vi "Type Query.vi"(8 "error in (no error)":errorcluster, 9 "Address (0)":i32, 11 "VISA resource name":refnum<visa-resource-name>) -> (0 "error out":errorcluster, 2 "Chamber Type":T1, 3 "VISA resource name out":refnum<visa-resource-name>)   [LabVIEW 2016, in "Environment Chamber.lvlib" / "Climatic Chamber.lvlib"]
doc: "<b>Chamber type monitor</B>\n\nReturns the type of sensor connected to the temperature controller, the type of temperature controller, and the set temperature upper limit."
uses:
  Climatic Chamber.lvlib
  Private/Type Defs/Chamber Type Cluster.ctl
  Private/Type Defs/Sensor Type Enum.ctl
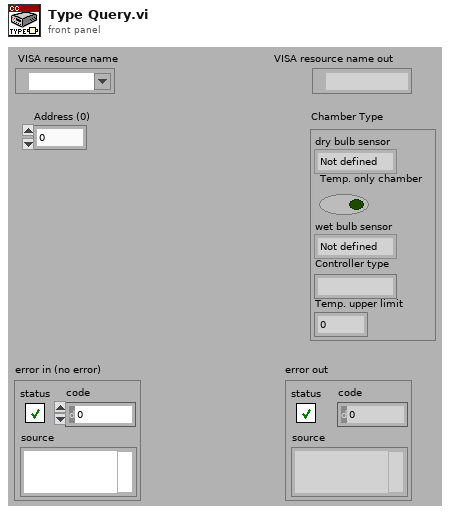
[diagram p1: front panel]
types:
  T1 = typedef "Environment Chamber.lvlib/Climatic Chamber.lvlib/Chamber Type Cluster.ctl" = cluster{"dry bulb sensor":T2, "Temp. only chamber":bool, "wet bulb sensor":T2, "Controller type":string, "Temp. upper limit":dbl}
  T2 = typedef "Environment Chamber.lvlib/Climatic Chamber.lvlib/Sensor Type Enum.ctl" = enum16{"Not defined", "Thermocouple"}
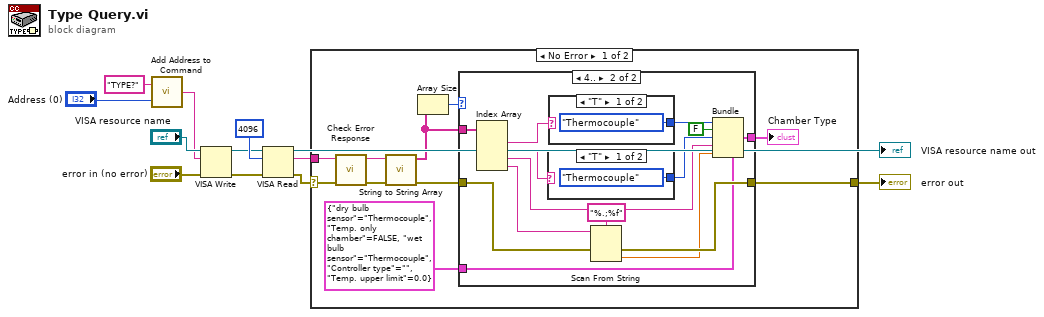
[diagram p0: block diagram]
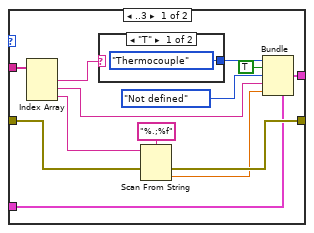
[diagram p2: hidden frame]
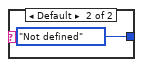
[diagram p3: hidden frame]
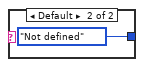
[diagram p4: hidden frame]
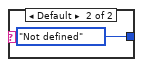
[diagram p5: hidden frame]
diagram:
  n1 = call "Add Address to Command.vi"("Address (0)"="Address (0)", "Command"="TYPE?") -> ("Command OUT"=w6:string)
  n2 = VISA Write(VISA resource name="VISA resource name", write buffer=w6, error in (no error)="error in (no error)") -> (VISA resource name out=w10:refnum<visa-resource-name>, error out=w9:errorcluster)  [unwired: 1 out]
  n3 = VISA Read(VISA resource name=w10, byte count=u32 4096 ("Bytes to Read"), error in (no error)=w9) -> (VISA resource name out=→"VISA resource name out":refnum<visa-resource-name>, read buffer=w3:string, error out=w2:errorcluster)  [unwired: 1 out]
  n4 = case shown="No Error" w2 {
    selector: w2 -> [w21 w56]
    tunnel: w3 -> [w22 _]
    tunnel: [w14 w56] -> w1
    frame No Error {
      n5 = call "Check Error Response.vi"("error in (no error)"=w21, "read String"=w22) -> ("error out"=w20:errorcluster, "String out"=w19:string)  [unwired: 7 in, 1 out]
      n6 = call "String to String Array.vi"("error in (no error)"=w20, "String received"=w19) -> ("error out"=w15:errorcluster, "Array Data"=w18:string[])  [unwired: 8 in]
      n7 = Array Size(array=w18) -> (size(s)=w17:i32)
      n8 = case shown="4.." w17 {
        tunnel: w18 -> [w34 w50]
        tunnel: T1 {"dry bulb sensor"=enum."Thermocouple", "Temp. only chamber"=FALSE, "wet bulb sensor"=enum."Thermocouple", "Controller type"="", "Temp. upper limit"=0.0} ("Chamber Type") -> [w31 w46]
        tunnel: w15 -> [w29 w41]
        tunnel: [w35 w51] -> w14
        tunnel: [w26 w38] -> w13
        frame ..3 {
          n9 = Index Array(array=w34) -> (element #1=w33:string, element #2=w25:string, element #3=w24:string)  [unwired: 3 in]
          n10 = case shown="\"T\"" w33 {
            tunnel: [Sensor_Type_Enum."Thermocouple" ("dry bulb sensor") Sensor_Type_Enum."Not defined" ("dry bulb sensor")] -> w32
            frame "T" {
            }
            frame Default {
            }
          }
          n11 = Scan From String(format string="%.;%f", input string=w24, error in=w29) -> (error out=w35:errorcluster, output 1=w28:dbl)  [unwired: 2 in, 2 out]
          n12 = Bundle(cluster=w31, "dry bulb sensor"=w32, "Temp. only chamber"=TRUE, "wet bulb sensor"=Sensor_Type_Enum."Not defined" ("dry bulb sensor"), "Controller type"=w25, "Temp. upper limit"=w28) -> (w26:T1)
        }
        frame 4.. {
          n13 = Index Array(array=w50) -> (element #1=w49:string, element #2=w48:string, element #3=w43:string, element #4=w42:string)  [unwired: 4 in]
          n14 = case shown="\"T\"" w48 {
            tunnel: [Sensor_Type_Enum."Thermocouple" ("dry bulb sensor") Sensor_Type_Enum."Not defined" ("dry bulb sensor")] -> w44
            frame "T" {
            }
            frame Default {
            }
          }
          n15 = case shown="\"T\"" w49 {
            tunnel: [Sensor_Type_Enum."Thermocouple" ("dry bulb sensor") Sensor_Type_Enum."Not defined" ("dry bulb sensor")] -> w47
            frame "T" {
            }
            frame Default {
            }
          }
          n16 = Scan From String(format string="%.;%f", input string=w42, error in=w41) -> (error out=w51:errorcluster, output 1=w40:dbl)  [unwired: 2 in, 2 out]
          n17 = Bundle(cluster=w46, "dry bulb sensor"=w47, "Temp. only chamber"=FALSE, "wet bulb sensor"=w44, "Controller type"=w43, "Temp. upper limit"=w40) -> (w38:T1)
        }
      }
      "Chamber Type" <- w13
    }
    frame Error {
    }
  }
  "error out" <- w1
